vi "Preserve Sent Message.vi"(8 "error in (no error)":errorcluster, 9 "Sent Message":string, 10 "To":string, 11 "Chat Window Model in":refnum<class "Chat Window Model.lvclass">) -> (0 "error out":errorcluster, 3 "Chat Window Model out":refnum<class "Chat Window Model.lvclass">)   [LabVIEW 2019, in "Chat Window Model.lvlib" / "Chat Window Model.lvclass"]
uses:
  Chat Window Model.lvclass
  Chat Window Model.lvclass/Chat Window Model.ctl
  Chat Window UI Controller/Chat Window UI Controller Messages/Update Message Window Msg/Update Message Window Msg.lvclass/Update Message Window Msg.ctl
  <vilib>/ActorFramework/Message Enqueuer/Message Enqueuer.lvclass/Message Enqueuer.ctl
  <vilib>/ActorFramework/Message Enqueuer/Enqueue.vi
  Chat Window UI Controller/Chat Window UI Controller Messages/Update Message Window Msg/Update Message Window Msg.lvclass
  C:/Program Files/National Instruments/LabVIEW 2019/vi.lib/ActorFramework/Message/Message.lvclass
  <vilib>/ActorFramework/Message Priority Queue/Priority Enqueue.vi
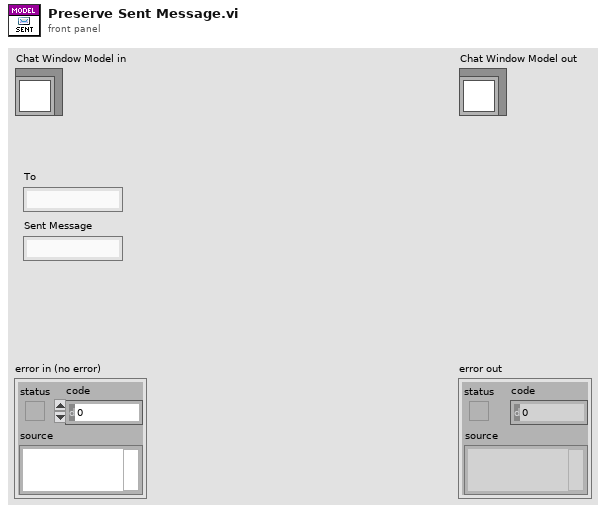
[diagram p1: front panel]
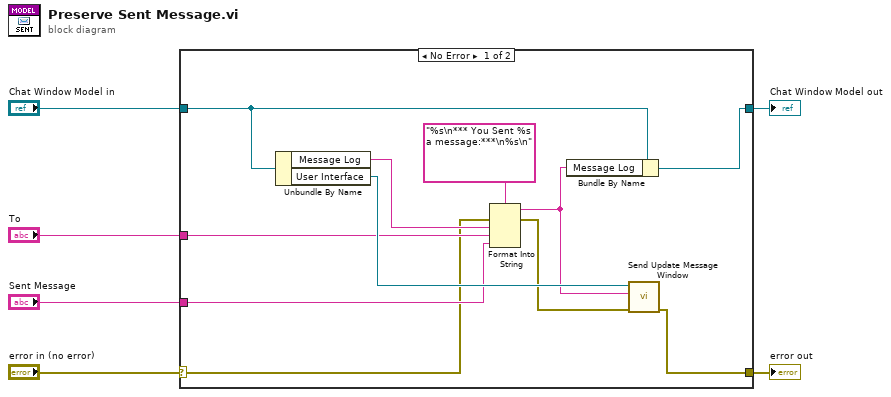
[diagram p0: block diagram]
diagram:
  n1 = case shown="No Error" "error in (no error)" {
    selector: "error in (no error)" -> [w8 w19]
    tunnel: [w7 w19] -> w5
    tunnel: [w13 w18] -> w3
    tunnel: "Chat Window Model in" -> [w12 w18]
    tunnel: "To" -> [w11 _]
    tunnel: "Sent Message" -> [w10 _]
    frame No Error {
      n2 = Unbundle By Name(w12) -> ("Message Log"=w15:string, "User Interface"=w17:refnum<class "Message Enqueuer.lvclass">)
      n3 = Format Into String(format string="%s\n*** You Sent %s a message:***\n%s\n", error in=w8, w15, w11, w10) -> (resulting string=w14:string, error out=w9:errorcluster)  [unwired: 1 in]
      n4 = Bundle By Name(cluster=w12, "Message Log"=w14) -> (w13:refnum<class "Chat Window Model.lvclass">)
      n5 = call "Send Update Message Window.vi"("error in (no error)"=w9, "Message"=w14, "Message Enqueuer"=w17) -> ("error out"=w7:errorcluster)  [unwired: 7 in, 1 out]
    }
    frame Error {
    }
  }
  "error out" <- w5
  "Chat Window Model out" <- w3
